vi "Get All PDO Communication Parameters.vi"(8 "error in":errorcluster, 9 "Type":enum16{"RX", "TX"}(ring), 10 "Node ID":u8, 11 "Obj Dict in":refnum<class "Object Dictionary.lvclass">) -> (0 "error out":errorcluster, 2 "PDO Communication Parameters":refnum<class "PDO Communication Parameter.lvclass">[](array[class]), 3 "Obj Dict out":refnum<class "Object Dictionary.lvclass">)   [LabVIEW 2020, in "CANopen.lvlib"]
uses:
  CANopen.lvlib
  Object Dictionary/Object Dictionary.lvclass
  PDO Communication Parameter/PDO Communication Parameter.lvclass
  RPDO Communication Parameter/RPDO Communication Parameter.lvclass
  D:/git/CANopen-LabVIEW/source/PDO Communication Parameter/PDO Communication Parameter.lvclass
  TPDO Communication Parameter/TPDO Communication Parameter.lvclass
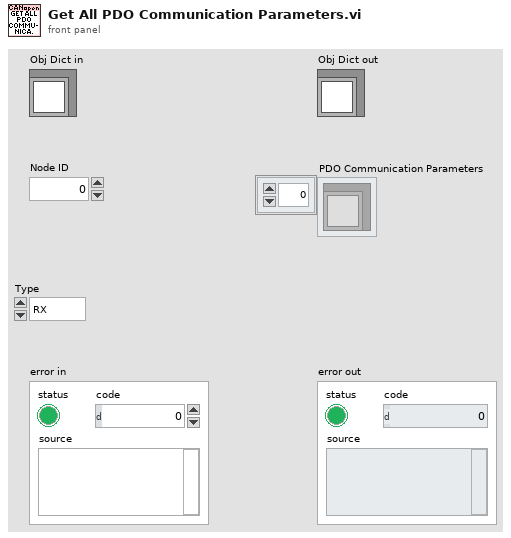
[diagram p1: front panel]
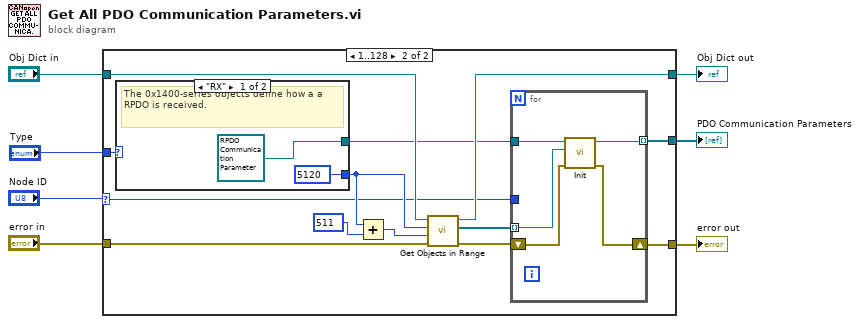
[diagram p0: block diagram]
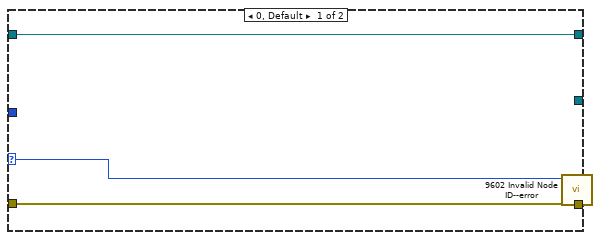
[diagram p2: hidden frame]
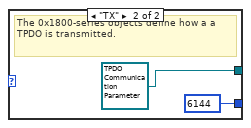
[diagram p3: hidden frame]
diagram:
  n1 = case shown="1..128" "Node ID" {
    selector: "Node ID" -> [w8 w14]
    tunnel: "error in" -> [w10 w24]
    tunnel: [w9 w22] -> w6
    tunnel: "Obj Dict in" -> [w11 w21]
    tunnel: [w11 w16] -> w4
    tunnel: "Type" -> [_ w15]
    tunnel: [_ w12] -> w1
    frame 0, Default {
      n2 = call "9602 Invalid Node ID--error.vi"("error in"=w10, "Node ID"=w8) -> ("error out"=w9:errorcluster)  [unwired: 8 in, 1 out]
    }
    frame 1..128 {
      n3 = case shown="\"RX\"" w15 {
        tunnel: [u16 5120 ("Start") u16 6144 ("Start")] -> w20
        tunnel: [refnum<class "RPDO Communication Parameter.lvclass"> refnum ("CANopen.lvlib:RX PDO Com Pam") refnum<class "TPDO Communication Parameter.lvclass"> refnum ("CANopen.lvlib:TX PDO Com Pam")] -> w13
        frame "RX" {
          # "The 0x1400-series objects define how a a RPDO is received."
        }
        frame "TX" {
          # "The 0x1800-series objects define how a a TPDO is transmitted."
        }
      }
      n4 = Add(x=w20, y=u16 511 ("Start")) -> (x+y=w18:u16)
      n5 = call "Get Objects in Range.vi"("error in"=w24, "End"=w18, "Start"=w20, "Obj Dict in"=w21) -> ("error out"=w23:errorcluster, "Objects in Range"=w17:refnum<class "Object Entry.lvclass">[], "Obj Dict out"=w16:refnum<class "Object Dictionary.lvclass">)  [unwired: 5 in]
      n6 = for {
        tunnel: [w25] -> w12 mode=indexing
        shift-right: [w26] -> w22
        shift-left: w23 -> [w27]
        tunnel: w17 -> [w28] mode=indexing
        tunnel: w14 -> [_]
        tunnel: w13 -> [w29]
        n7 = call-dynamic "Init.vi"("error in"=w27, "OD Entry"=w28, "PDO Communication Parameter in"=w29) -> ("error out"=w26:errorcluster, "PDO Communication Parameter out"=w25:refnum<class "PDO Communication Parameter.lvclass">)  [unwired: 7 in]
      }
    }
  }
  "Obj Dict out" <- w4
  "error out" <- w6
  "PDO Communication Parameters" <- w1
